vi "Actor Core.vi"(8 "error in":errorcluster, 11 "Nested in":refnum<class "BD Protocol 4.0.lvclass">) -> (0 "error out":errorcluster, 3 "Actor out":refnum<class "Actor.lvclass">)   [LabVIEW 2016, in "BD Protocol 4.0.lvlib" / "BD Protocol 4.0.lvclass"]
doc: "(<B>Filename</B>: Actor Framework.lvlib:Actor.lvclass:Actor Core.vi)\n\nReceives messages to the actor, reacts to them, and initiates any error handling that may shut the actor down.\n\nDescendant classes may override this VI to append parallel tasks for the actor to complete while it handles messages. Overrides use the Call Parent Method node."
uses:
  BD Protocol 4.0.lvclass
  C:/Program Files (x86)/National Instruments/LabVIEW 2016/vi.lib/ActorFramework/Actor/Actor.lvclass
  <vilib>/ActorFramework/Actor/Actor.lvclass
  BD Protocol 4.0.lvclass/BD Protocol 4.0.ctl
  <vilib>/ActorFramework/Actor/Actor.lvclass/Actor.ctl
  <vilib>/ActorFramework/Message Enqueuer/Message Enqueuer.lvclass/Message Enqueuer.ctl
  <vilib>/ActorFramework/Message Enqueuer/Init from Existing Queue.vi
  <vilib>/ActorFramework/Message Enqueuer/Enqueue.vi
  C:/Program Files (x86)/National Instruments/LabVIEW 2016/vi.lib/ActorFramework/Message/Message.lvclass
  <vilib>/ActorFramework/Stop Msg/Stop Msg.lvclass
  <vilib>/ActorFramework/Message Priority Queue/Priority Enqueue.vi
  <vilib>/ActorFramework/Message Enqueuer/Message Enqueuer.lvclass
panel:
  out "Decode Data":string
  out "Raw Data":string
  out "Serial port status":bool
  in  "打开":bool
  in  "baud rate":u32(ring)=115200 caption="波特率" items=["4800"=4800, "9600"=9600, "19200"=19200, "38400"=38400, "115200"=115200]
  in  "Serial port":refnum<visa-resource-name> caption="串口"
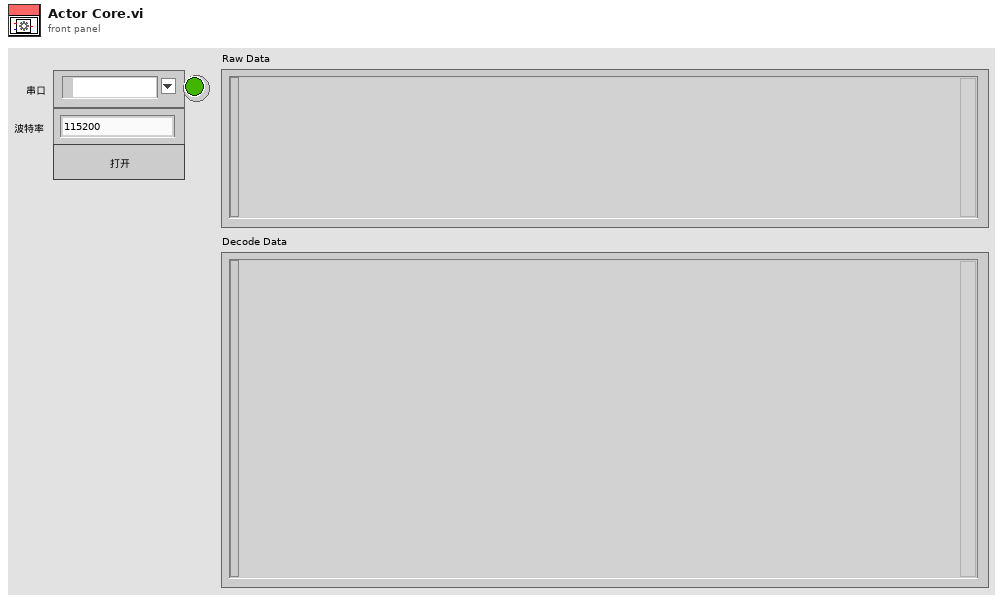
[diagram p1: front panel]
types:
  T1 = cluster{"Stop":refnum<user-event>, "Serial port status":refnum<user-event>, "Raw Data":refnum<user-event>, "Decode Data":refnum<user-event>}
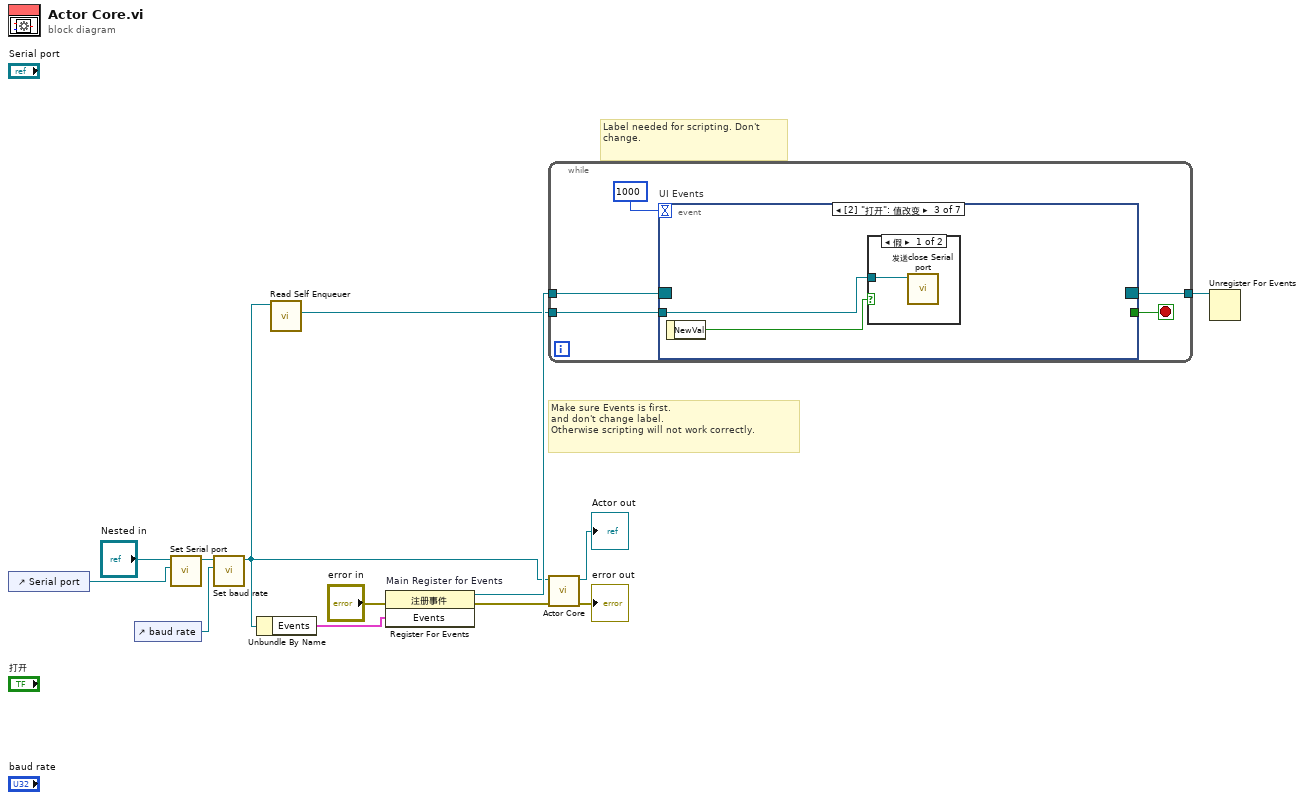
[diagram p0: block diagram]
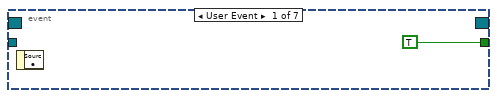
[diagram p2: hidden frame]
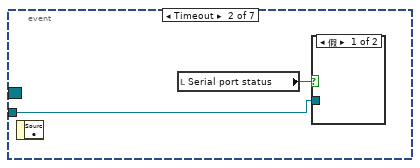
[diagram p3: hidden frame]
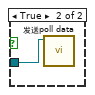
[diagram p4: hidden frame]
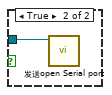
[diagram p5: hidden frame]
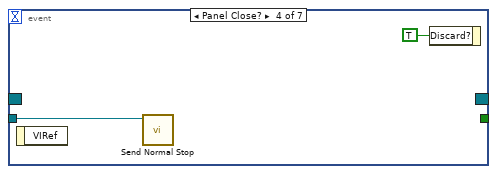
[diagram p6: hidden frame]
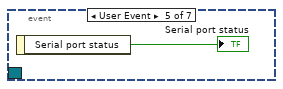
[diagram p7: hidden frame]
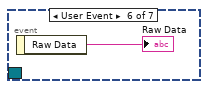
[diagram p8: hidden frame]
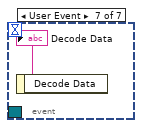
[diagram p9: hidden frame]
diagram:
  # "Label needed for scripting. Don't change."
  # "Make sure Events is first.\nand don't change label.\nOtherwise scripting will not work correctly."
  n1 = control-ref of="Serial port"() -> (w4:refnum<vi>)
  n2 = control-ref of="baud rate"() -> (w3:refnum<vi>)
  n3 = call "Set Serial port.vi"("Serial port"=w4, "BD Protocol 4.0 in"="Nested in") -> ("BD Protocol 4.0 out"=w5:refnum<class "BD Protocol 4.0.lvclass">)  [unwired: 9 in]
  n4 = call "Set baud rate.vi"("baud rate"=w3, "BD Protocol 4.0 in"=w5) -> ("BD Protocol 4.0 out"=w1:refnum<class "BD Protocol 4.0.lvclass">)  [unwired: 9 in]
  n5 = Unbundle By Name(w1) -> ("Events"=w10:T1)
  n6 = call <vilib>:"Read Self Enqueuer.vi"("Actor"=w1) -> ("Self Enqueuer"=w8:refnum<class "Message Enqueuer.lvclass">)  [unwired: 10 in]
  n7 = register-events "Main Register for Events"(error in="error in", w10) -> (reference out=w11:refnum<event-registration>, error out=w6:errorcluster)  [unwired: 1 in]
  n8 = while {
    tunnel: w11 -> [w18]
    tunnel: [w16] -> w9
    tunnel: w8 -> [w15]
    stop <- w17 stop-if-true
    n9 = event "UI Events" shown="[2] \"打开\": 值改变" {
      selector: w18 -> [_ _ _ _ _ _ _]
      dyn-events: [_ _ _ _ _ _ _] -> w16
      timeout: 1000 -> [_ _ _ _ _ _ _]
      tunnel: [TRUE _ _ _ _ _ _] -> w17
      tunnel: w15 -> [_ w21 w23 w27 _ _ _]
      event User Event {
        n10 = event-data() -> ()  [unwired: 1 in, 1 out]
      }
      event Timeout {
        n11 = event-data() -> ()  [unwired: 1 in, 1 out]
        n12 = local read "Serial port status"() -> (w20:bool)
        n13 = case shown="假" w20 {
          tunnel: w21 -> [_ w22]
          frame False {
          }
          frame True {
            n14 = call "发送poll data.vi"("Message Enqueuer"=w22) -> ()  [unwired: 9 in, 2 out]
          }
        }
      }
      event "打开": Value Change {
        n15 = event-data() -> ("NewVal"=w24:bool)  [unwired: 1 in]
        n16 = case shown="假" w24 {
          tunnel: w23 -> [w25 w26]
          frame False {
            n17 = call "发送close Serial port.vi"("Message Enqueuer"=w25) -> ()  [unwired: 9 in, 2 out]
          }
          frame True {
            n18 = call "发送open Serial port.vi"("Message Enqueuer"=w26) -> ()  [unwired: 9 in, 2 out]
          }
        }
      }
      event Panel Close? {
        n19 = event-data() -> ()  [unwired: 1 in, 1 out]
        n20 = call <vilib>:"Send Normal Stop.vi"("Message Enqueuer"=w27) -> ()  [unwired: 10 in, 1 out]
        n21 = event-data("Discard?"=TRUE) -> ()  [unwired: 1 in, 1 out]
      }
      event User Event {
        n22 = event-data() -> ("Serial port status"=→"Serial port status":bool)  [unwired: 1 in]
      }
      event User Event {
        n23 = event-data() -> ("Raw Data"=→"Raw Data":string)  [unwired: 1 in]
      }
      event User Event {
        n24 = event-data() -> ("Decode Data"=→"Decode Data":string)  [unwired: 1 in]
      }
    }
  }
  n25 = call-parent "Actor Core.vi"("error in"=w6, "Actor in"=w1) -> ("error out"=→"error out":errorcluster, "Actor out"=→"Actor out":refnum<class "Actor.lvclass">)  [unwired: 8 in]
  n26 = Unregister For Events(event registration refnum=w9) -> ()  [unwired: 1 in, 1 out]
